vi "Add Headers.vi"(8 "error in (no error)":errorcluster, 10 "Headers":T1[](array[typedef]), 11 "REST_Client in":refnum<class "REST_Client.lvclass">) -> (0 "error out":errorcluster, 3 "REST_Client out":refnum<class "REST_Client.lvclass">)   [LabVIEW 2020, in "REST_Client.lvclass"]
uses:
  REST_Client.lvclass
  <vilib>/httpClient/LabVIEWHTTPClient.lvlib
  Header Info.ctl
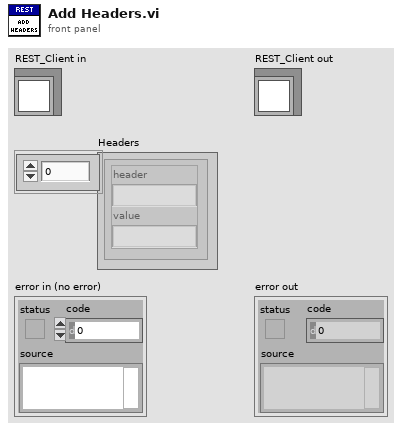
[diagram p1: front panel]
types:
  T1 = typedef "REST_Client.lvclass/Header Info.ctl" = cluster{"header":string, "value":string}
  T2 = typedef "LabVIEWHTTPClient.lvlib/ClientHandle.ctl" = refnum<k1>
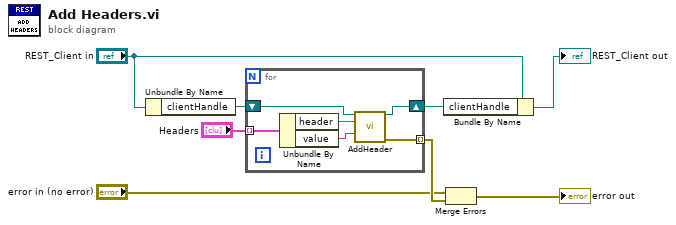
[diagram p0: block diagram]
diagram:
  n1 = Unbundle By Name("REST_Client in") -> ("clientHandle"=w7:T2)
  n2 = for {
    tunnel: "Headers" -> [w12] mode=indexing
    shift-right: [w10] -> w5
    shift-left: w7 -> [w11]
    tunnel: [w9] -> w3 mode=indexing
    n3 = Unbundle By Name(w12) -> ("header"=w14:string, "value"=w13:string)
    n4 = call <vilib>:"AddHeader.vi"("client handle"=w11, "header"=w14, "value"=w13) -> ("client handle out"=w10:T2, "error out"=w9:errorcluster)  [unwired: 11 in]
  }
  n5 = Bundle By Name(cluster="REST_Client in", "clientHandle"=w5) -> (→"REST_Client out":refnum<class "REST_Client.lvclass">)
  n6 = Merge Errors("error in (no error)", w3) -> (→"error out":errorcluster)
